vi "GetFirstFreeObsolete.vi"(8 "error in (no error)":errorcluster, 10 "LibraryName":string, 11 "Connection in":refnum<class "Connection.lvclass">) -> (0 "error out":errorcluster, 1 "FirstFreeObsolete":i32, 2 "Valid":bool, 3 "Connection out":refnum<class "Connection.lvclass">)   [LabVIEW 2021, in "ErrorDefinitionSQLite.lvclass"]
uses:
  ErrorDefinitionSQLite.lvclass
  <vilib>/drjdpowell/SQLite Library/SQL Connection/Connection.lvclass
  <vilib>/drjdpowell/SQLite Library/SQL Connection/Execute SQL.vi
  <vilib>/drjdpowell/SQLite Library/SQLite.lvlib
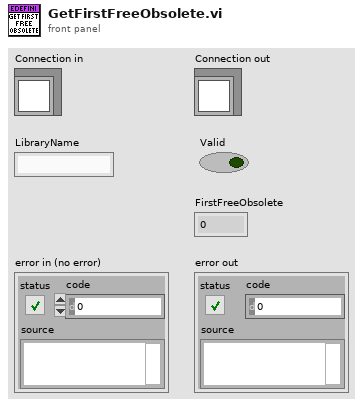
[diagram p1: front panel]
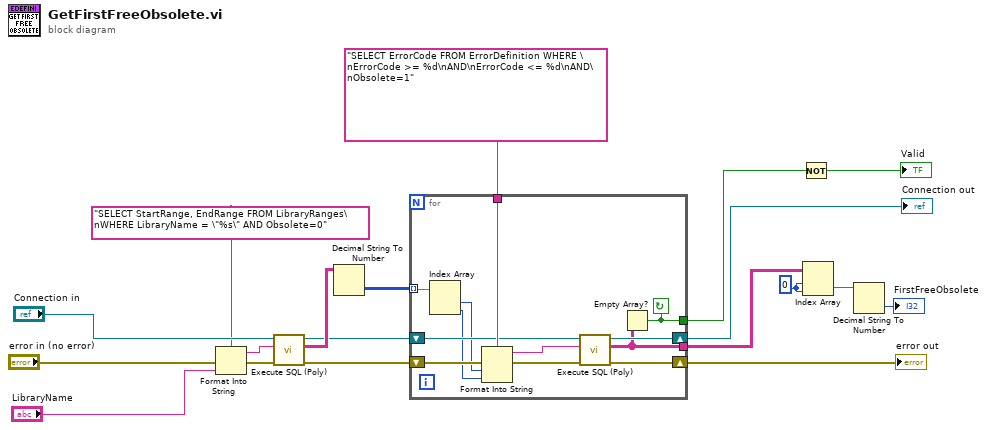
[diagram p0: block diagram]
diagram:
  w2 = 0 ("index (row)")
  n1 = Format Into String(format string="SELECT StartRange, EndRange FROM LibraryRanges\nWHERE LibraryName = \"%s\" AND Obsolete=0" ("SQL"), error in="error in (no error)", "LibraryName") -> (resulting string=w17:string, error out=w14:errorcluster)  [unwired: 1 in]
  n2 = call-poly <vilib>:"Execute SQL (Poly).vi"("error in (no error)"=w14, "SQL"=w17, "SQLite Connection in"="Connection in") -> ("error out"=w15:errorcluster, "Result Set"=w18:string[][], "SQLite Connection"=w16:refnum<class "Connection.lvclass">)  [unwired: 5 in, 1 out]
  n3 = Decimal String To Number(string=w18) -> (number=w19:i32[][])  [unwired: 2 in, 1 out]
  n4 = for {
    tunnel: [w28] -> w3
    tunnel: [w20] -> w7
    tunnel: "SELECT ErrorCode FROM ErrorDefinition WHERE \nErrorCode >= %d\nAND\nErrorCode <= %d\nAND\nObsolete=1" ("SQL") -> [w26]
    shift-right: [w27] -> w8
    shift-left: w15 -> [w25]
    shift-right: [w29] -> w6
    shift-left: w16 -> [w24]
    tunnel: w19 -> [w23] mode=indexing
    stop <- w20 continue-if-true
    n5 = Index Array(array=w23) -> (element #1=w22:i32, element #2=w21:i32)  [unwired: 2 in]
    n6 = Format Into String(format string=w26, error in=w25, w22, w21) -> (resulting string=w30:string, error out=w31:errorcluster)  [unwired: 1 in]
    n7 = call-poly <vilib>:"Execute SQL (Poly).vi"("error in (no error)"=w31, "SQL"=w30, "SQLite Connection in"=w24) -> ("error out"=w27:errorcluster, "Result Set"=w28:string[][], "SQLite Connection"=w29:refnum<class "Connection.lvclass">)  [unwired: 5 in, 1 out]
    n8 = Empty Array?(array=w28) -> (empty?=w20:bool)
  }
  "error out" <- w8
  "Connection out" <- w6
  n9 = Not(x=w7) -> (.not. x?=→"Valid":bool)
  n10 = Index Array(array=w3, index (row)=w2, index (col)=w2) -> (element=w5:string)
  n11 = Decimal String To Number(string=w5) -> (number=→"FirstFreeObsolete":i32)  [unwired: 2 in, 1 out]
